vi "Main.vi"(8 "error in (no error)":errorcluster, 11 "ModuleAdmin":refnum<class "ModuleAdmin.lvclass">) -> ()   [LabVIEW 2018, in "SensorModule.lvlib"]
uses:
  SensorModule.lvlib
  <userlib>/NIST/ModuleAdminLib/ModuleAdmin/ModuleAdmin.lvclass
  C:/Program Files (x86)/National Instruments/LabVIEW 2018/user.lib/NIST/ModuleAdminLib/ModuleAdminBase/ModuleAdminBase.lvclass
  SensorPlugins/SensorBaseClass/SensorBase.lvclass
  C:/Program Files (x86)/National Instruments/LabVIEW 2018/user.lib/NIST/BaseClasses/BasePlugin_class/BasePlugin.lvclass
  PublicAPI/Arguments/Requests/clStopArgument.ctl
  <userlib>/NIST/ModuleAdminLib/ModuleAdmin/ModuleAdmin.lvclass/ModuleAdmin.ctl
  <userlib>/NIST/BaseClasses/BasePlugin_class/BasePlugin.lvclass/BasePlugin.ctl
  <vilib>/Utility/error.llb/DialogType.ctl
  <userlib>/NIST/ModuleAdminLib/ModuleAdmin/Accessors/Read ShowPanel_.vi
  <userlib>/NIST/ModuleAdminLib/ModuleAdmin/Accessors/Write ShowPanel_.vi
  <userlib>/NIST/BaseClasses/BasePlugin_class/Accessors/Write PluginIniFilePath.vi
  <userlib>/NIST/BaseClasses/BasePlugin_class/Accessors/Read PluginIniFilePath.vi
  <userlib>/NIST/ModuleAdminLib/ModuleAdmin/Accessors/Read CloneRegRef.vi
  <vilib>/Utility/error.llb/Error Cluster From Error Code.vi
  <vilib>/ErrorRing/Error Ring.xnode
  <userlib>/NIST/ModuleAdminLib/CloneRegistration/CloneRegistration.lvclass
  <userlib>/NIST/BaseClasses/Object_class/BaseObject.lvclass
  <userlib>/NIST/ModuleAdminLib/ModuleAdmin.lvlib
panel:
  out "error out":errorcluster
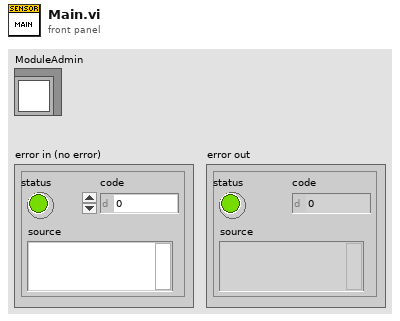
[diagram p1: front panel]
types:
  T1 = typedef "SensorModule.lvlib/clRequestEvents.ctl" = cluster{"StopRequest":refnum<user-event>, "PathToINI":refnum<user-event>, " LoadPlugin":refnum<user-event>, "ShowPanel":refnum<user-event>, "StartData":refnum<user-event>, "StopData":refnum<user-event>, "WriteConfig":refnum<user-event>, "ReadConfig":refnum<user-event>, "WriteEvtSignal":refnum<user-event>, "Configure":refnum<user-event>}
  T2 = typedef "SensorModule.lvlib/clBroadcastEvents.ctl" = cluster{"DidInit":refnum<user-event>, "StatusUpdate":refnum<user-event>, "ErrorReport":refnum<user-event>, "DidStop":refnum<user-event>, "PathToINI":refnum<user-event>, "SensorReport":refnum<user-event>, "SensorConfig":refnum<user-event>}
  T3 = typedef "SensorModule.lvlib/clStopArgument.ctl" = cluster{"Exit via Stop Module Req?":bool, "Wait for Module to stop?":bool, "ModuleAdmin":refnum<class "ModuleAdmin.lvclass">}
  T4 = enum32{"Invalid", "Standard", "Closed", "Hidden", "Minimized", "Maximized"}
  T5 = typedef "SensorModule.lvlib/clSensorData.ctl" = cluster{"SensorType":string, "SensorData":variant}
  T6 = typedef "DialogType.ctl" = u16
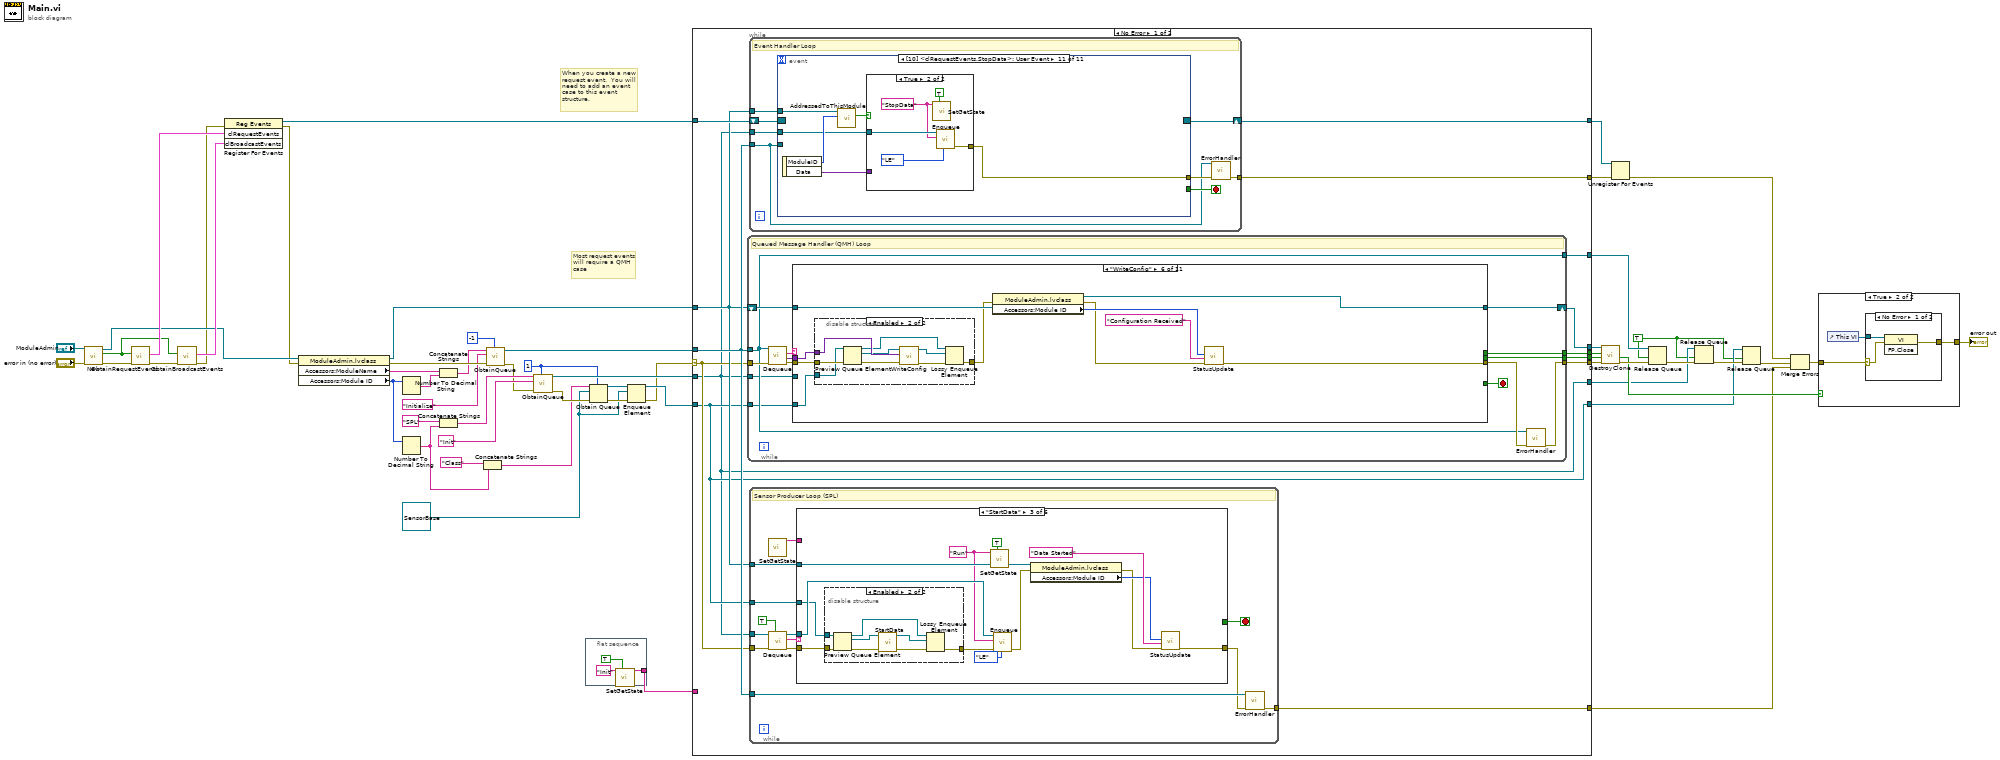
[diagram p0: block diagram]
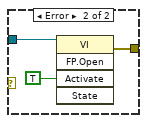
[diagram p3: hidden frame]
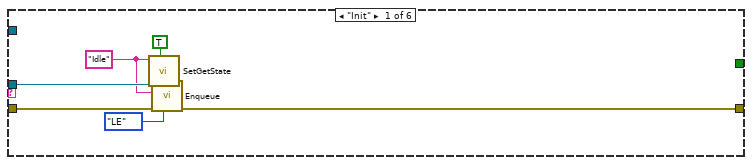
[diagram p4: hidden frame]
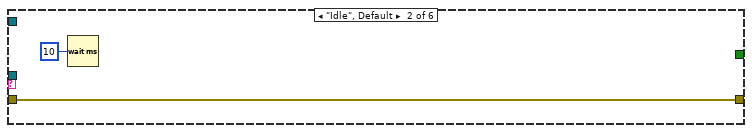
[diagram p5: hidden frame]
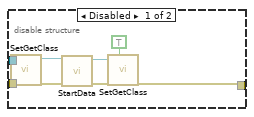
[diagram p6: hidden frame]
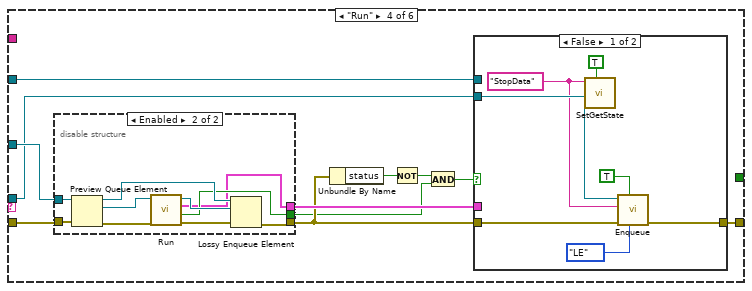
[diagram p7: hidden frame]
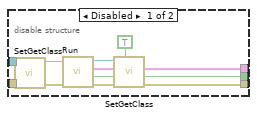
[diagram p8: hidden frame]
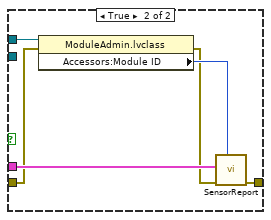
[diagram p9: hidden frame]
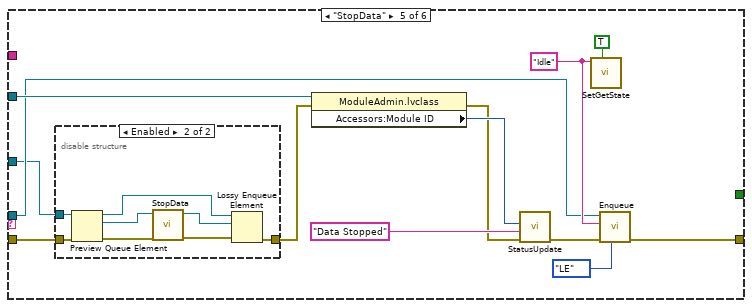
[diagram p10: hidden frame]
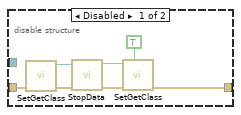
[diagram p11: hidden frame]
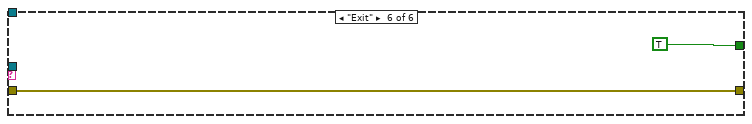
[diagram p12: hidden frame]
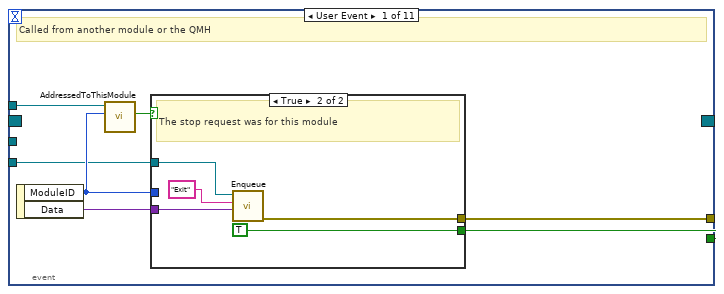
[diagram p13: hidden frame]
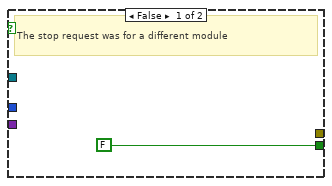
[diagram p14: hidden frame]
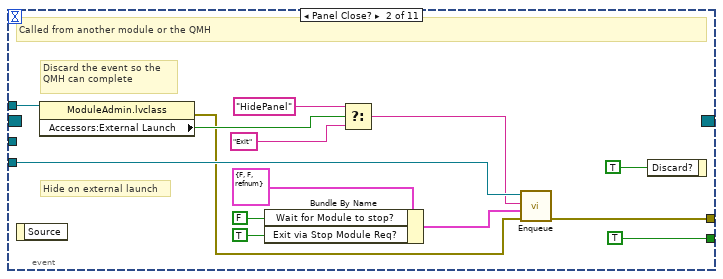
[diagram p15: hidden frame]
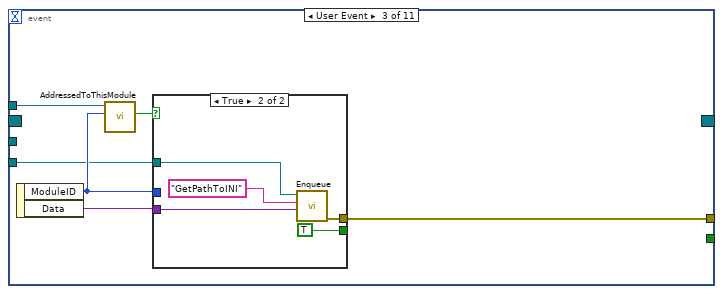
[diagram p16: hidden frame]
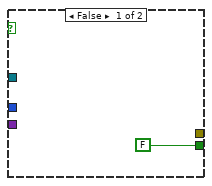
[diagram p17: hidden frame]
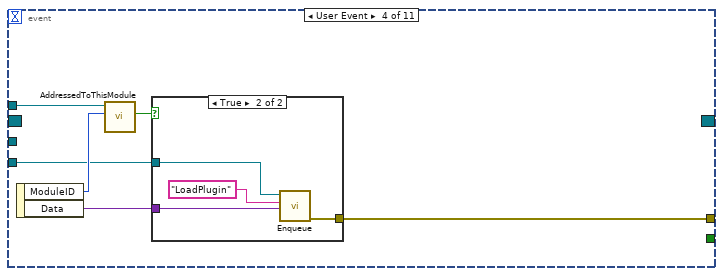
[diagram p18: hidden frame]
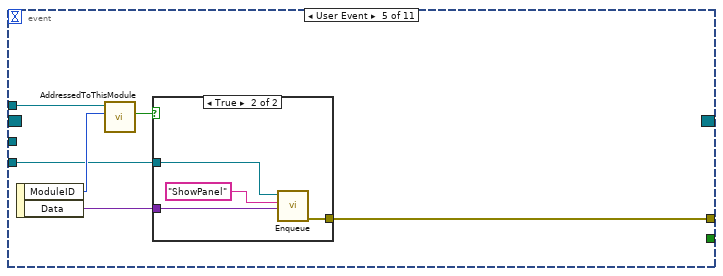
[diagram p20: hidden frame]
diagram:
  w2 = TRUE ("force destroy? (F)")
  w11 = refnum<class "SensorBase.lvclass"> refnum ("MyPlugins.lvlib:MyPluginsBase.lvclass")
  w1 = 1 ("Queue size (-1, unlimited)")
  # "Most request events\nwill require a QMH\ncase"
  # "When you create a new request event.  You will need to add an event case to this event structure."
  n1 = call <userlib>:"New.vi"("error in (no error)"="error in (no error)", "ModuleAdmin"="ModuleAdmin") -> ("error out"=w53:errorcluster, "First?"=w49:bool, "ModuleAdmin"=w34:refnum<class "ModuleAdmin.lvclass">)  [unwired: 6 in, 1 out]
  n2 = call "ObtainRequestEvents.vi"("error in (no error)"=w53, "CreateNew (F)"=w49) -> ("error out"=w48:errorcluster, "clRequestEvents"=w52:T1)  [unwired: 8 in]
  n3 = call "ObtainBroadcastEvents.vi"("error in (no error)"=w48, "CreateNew? (F)"=w49) -> ("error out"=w21:errorcluster, "clBroadcastEvents"=w47:T2)  [unwired: 8 in]
  n4 = register-events(error in=w21, w52, w47) -> (reference out=w46:refnum<event-registration>, error out=w20:errorcluster)  [unwired: 1 in]
  n5 = property class="ModuleAdmin.lvclass"(reference=w34, error in=w20) -> (reference out=w8:refnum<class "ModuleAdmin.lvclass">, error out=w36:errorcluster, "Accessors:ModuleName"=w32:string, "Accessors:Module ID"=w24:i32)
  n6 = Number To Decimal String(number=w24) -> (decimal integer string=w31:string)  [unwired: 1 in]
  n7 = Number To Decimal String(number=w24) -> (decimal integer string=w15:string)  [unwired: 1 in]
  n8 = Concatenate Strings(w32, w31) -> (w30:string)
  n9 = Concatenate Strings("SPL" ("Initial Message"), w15) -> (w26:string)
  n10 = Concatenate Strings("Class" ("Initial Message"), w15) -> (w14:string)
  n11 = call "ObtainQueue.vi"("Queue size (-1, unlimited)"=-1, "error in (no error)"=w36, "Initial Message"="Initialize", "Queue Name"=w30) -> ("error out"=w25:errorcluster, "MessageQueue"=w51:refnum<queue>)  [unwired: 6 in]
  n12 = call "ObtainQueue.vi"("Queue size (-1, unlimited)"=w1, "error in (no error)"=w25, "Initial Message"="Init", "Queue Name"=w26) -> ("error out"=w18:errorcluster, "MessageQueue"=w22:refnum<queue>)  [unwired: 6 in]
  n13 = flat-sequence {
    tunnel: [w56] -> w9
    frame #0 {
      n14 = call "SetGetState.vi"("Set (f)"=TRUE, "State In"="Init") -> ("State Out"=w56:string)  [unwired: 9 in]
    }
  }
  n15 = Obtain Queue(max queue size (-1, unlimited)=w1, name (unnamed)=w14, element data type=w11, error in (no error)=w18) -> (queue out=w13:refnum<queue>, error out=w17:errorcluster)  [unwired: 1 in, 1 out]
  n16 = Enqueue Element(queue=w13, element=w11, error in (no error)=w17) -> (queue out=w12:refnum<queue>, error out=w10:errorcluster)  [unwired: 1 in, 1 out]
  n17 = case shown="No Error" w10 {
    selector: w10 -> [w61 w618]
    tunnel: w51 -> [w65 w614]
    tunnel: w8 -> [w63 w615]
    tunnel: [w72 w616] -> w45
    tunnel: [w71 w614] -> w50
    tunnel: w46 -> [w70 w610]
    tunnel: [w69 w613] -> w43
    tunnel: [w68 _] -> w42
    tunnel: [w67 _] -> w41
    tunnel: [w66 _] -> w39
    tunnel: [w64 _] -> w19
    tunnel: [w62 w610] -> w38
    tunnel: w22 -> [w59 w607]
    tunnel: w12 -> [w60 w606]
    tunnel: w9 -> [_ _]
    tunnel: [w59 w607] -> w4
    tunnel: [w60 w606] -> w3
    frame No Error {
      n18 = while {
        tunnel: w65 -> [w321]
        tunnel: w61 -> [w330]
        tunnel: [w323] -> w72
        tunnel: [w321] -> w71
        tunnel: [w325] -> w68
        tunnel: [w324] -> w67
        shift-right: [w320] -> w69
        shift-left: w63 -> [w326]
        tunnel: w60 -> [w319]
        tunnel: w59 -> [w318]
        stop <- w331 stop-if-true
        # "Queued Message Handler (QMH) Loop"
        n19 = call "Dequeue.vi"("error in (no error)"=w330, "MessageQueue"=w321) -> ("error out"=w329:errorcluster, "Message Data"=w327:variant, "Message"=w328:string)  [unwired: 6 in, 1 out]
        n20 = case shown="\"WriteConfig\"" w328 {
          selector: w328 -> [_ _ _ _ _ _ _ _ _ _ w594]
          tunnel: [_ _ _ _ _ _ _ _ w562 _ _] -> w331
          tunnel: w326 -> [w354 w371 w378 w448 w463 w493 w517 w539 w563 w572 w597]
          tunnel: [w343 w365 w379 w449 w462 w491 w513 w537 w557 w573 w588] -> w322
          tunnel: w329 -> [w332 w374 w388 w446 w464 w487 w519 w533 w559 w570 w591]
          tunnel: w327 -> [_ w373 w390 _ _ w488 _ w534 w567 w580 _]
          tunnel: [_ _ _ _ _ _ _ _ w565 _ _] -> w325
          tunnel: [_ _ _ _ _ _ _ _ w564 _ _] -> w324
          tunnel: [w336 w370 w376 w445 w463 w492 w512 w538 w563 w568 w592] -> w320
          tunnel: w319 -> [_ _ w375 w442 w461 w484 w509 w530 _ _ _]
          tunnel: w318 -> [_ _ _ _ _ _ _ _ w561 _ _]
          frame "Initialize" {
            # "Initialize is always called after ObtainQueue.vi is run"
            n21 = property class="ModuleAdmin.lvclass"(reference=w354, error in=w332) -> (reference out=w341:refnum<class "ModuleAdmin.lvclass">, error out=w351:errorcluster, "Accessors:Module ID"=w333:i32, "Accessors:ShowPanel_"=w339:bool, "Accessors:External Launch"=w338:bool, "Accessors:ModuleName"=w340:string)
            n22 = call "SetGetClass.vi"("Set (f)"=TRUE, "Class In"=refnum<class "SensorBase.lvclass"> refnum ("MyPlugins.lvlib:MyPluginsBase.lvclass")) -> ()  [unwired: 9 in, 1 out]
            n23 = Compound Arithmetic op=OR(w339, invert w338) -> (w337:bool)
            n24 = Select(t=T4."Standard" ("Front Panel Window:State"), s=w337, f=T4."Hidden" ("Front Panel Window:State")) -> (s? t:f=w347:T4)
            n25 = invoke class="VI" method="FP.Open"(error in=w351, "State"=w347) -> (error out=w350:errorcluster)  [unwired: 3 in, 4 out]
            n26 = call <userlib>:"ModuleName.vi"("Name"=w340, "ModuleID"=w333) -> ("ModuleName"=w346:string)  [unwired: 9 in]
            n27 = property class="VI"(error in=w350, "Front Panel.Title"=w346) -> (reference out=w353:refnum<vi>, error out=w352:errorcluster)  [unwired: 1 in]
            n28 = invoke class="VI" method="FP.Center"(reference=w353, error in=w352) -> (error out=w342:errorcluster)  [unwired: 1 in, 2 out]
            n29 = case shown="True" w338 {
              tunnel: [w355 w361] -> w344
              tunnel: [w356 w358] -> w336
              tunnel: w342 -> [w355 w360]
              tunnel: w341 -> [w356 w357]
              frame False {
              }
              frame True {
                n30 = call <userlib>:"WaitOnModuleSync.vi"("error in (no error)"=w360, "ModuleAdmin"=w357) -> ("error out"=w362:errorcluster, "ModuleAdmin"=w359:refnum<class "ModuleAdmin.lvclass">)  [unwired: 8 in]
                n31 = call <userlib>:"WaitOnEventSync.vi"("error in (no error)"=w362, "ModuleAdmin"=w359) -> ("error out"=w361:errorcluster, "ModuleAdmin"=w358:refnum<class "ModuleAdmin.lvclass">)  [unwired: 8 in]
              }
            }
            n32 = call "DidInit.vi"("Init?"=TRUE, "error in (no error)"=w344, "ModuleAdmin"=w336) -> ("error out"=w343:errorcluster)  [unwired: 8 in]
          }
          frame "ShowPanel" {
            n33 = Variant To Data(error in=w374, type=TRUE, Variant=w373) -> (data=w367:bool, error out=w364:errorcluster)
            n34 = property class="ModuleAdmin.lvclass"(reference=w371, error in=w364, "Accessors:ShowPanel_"=w367) -> (reference out=w370:refnum<class "ModuleAdmin.lvclass">, error out=w363:errorcluster)
            n35 = Select(t=T4."Standard" ("Front Panel Window:State"), s=w367, f=T4."Hidden" ("Front Panel Window:State")) -> (s? t:f=w366:T4)
            n36 = property class="VI"(error in=w363, "FP.State"=w366) -> (error out=w365:errorcluster)  [unwired: 1 in, 1 out]
          }
          frame "LoadPlugin" {
            n37 = Variant To Data(error in=w388, type=path "", Variant=w390) -> (data=w377:path, error out=w387:errorcluster)
            n38 = Current VI's Path() -> (path=w385:path)
            n39 = call <userlib>:"GetPathToClass.vi"("error in (no error)"=w387, "configuration file path"=w377) -> ("error IO"=w383:errorcluster, "PathToClass"=w386:path)  [unwired: 8 in]
            n40 = Build Path(base path=w385, name or relative path=w386) -> (appended path=w384:path)
            n41 = call <vilib>:"Check if File or Folder Exists.vi"("error in (no error)"=w383, "path"=w384) -> ("error out"=w380:errorcluster, "file or folder exists?"=w382:bool, "dup path"=w381:path)  [unwired: 7 in]
            n42 = case shown="False" w382 {
              tunnel: w381 -> [w393 w404]
              tunnel: w380 -> [_ w416]
              tunnel: [w392 w407] -> w379
              tunnel: w378 -> [w391 w412]
              tunnel: w377 -> [_ w410]
              tunnel: [w391 w409] -> w376
              tunnel: w375 -> [_ w402]
              frame False {
                n43 = Path To String(path=w393) -> (string=w394:string)
                n44 = xnode "Error Ring"("parameter 0"=w394) -> ("error out"=w392:errorcluster)
              }
              frame True {
                n45 = disable-structure shown="Enabled" {
                  disable-tunnel: w416 -> [w427 w435]
                  disable-tunnel: w410 -> [w423 w439]
                  disable-tunnel: [w418 w429] -> w406
                  disable-tunnel: w404 -> [w417 w436]
                  disable-tunnel: [w417 w436] -> w403
                  disable-tunnel: w402 -> [_ w432]
                  frame Disabled {
                    n46 = call-dynamic "LoadClassFromFile.vi"("error in (no error)"=w427, "class path"=w417, "reference in"=refnum<class "SensorBase.lvclass"> refnum ("MyPlugins.lvlib:MyPluginsBase.lvclass")) -> ("error out"=w424:errorcluster, "reference out"=w425:refnum<class "SensorBase.lvclass">)  [unwired: 7 in]
                    n47 = property class="SensorBase.lvclass"(reference=w425, error in=w424, "Accessors:PluginIniFilePath"=w423) -> (reference out=w421:refnum<class "SensorBase.lvclass">, error out=w419:errorcluster)
                    n48 = call-dynamic "DefaultFromIni.vi"("error in (no error)"=w419, "SensorBase in"=w421) -> ("error out"=w418:errorcluster, "SensorBase out"=w420:refnum<class "SensorBase.lvclass">)  [unwired: 8 in]
                    n49 = call "SetGetClass.vi"("Set (f)"=TRUE, "Class In"=w420) -> ()  [unwired: 9 in, 1 out]
                  }
                  frame Enabled {
                    n50 = Preview Queue Element(queue=w432, error in (no error)=w435) -> (queue out=w428:refnum<queue>, element=w433:refnum<class "SensorBase.lvclass">, error out=w434:errorcluster)  [unwired: 1 in, 1 out]
                    n51 = call-dynamic "LoadClassFromFile.vi"("error in (no error)"=w434, "class path"=w436, "reference in"=w433) -> ("error out"=w440:errorcluster, "reference out"=w441:refnum<class "SensorBase.lvclass">)  [unwired: 7 in]
                    n52 = property class="SensorBase.lvclass"(reference=w441, error in=w440, "Accessors:PluginIniFilePath"=w439) -> (reference out=w438:refnum<class "SensorBase.lvclass">, error out=w437:errorcluster)
                    n53 = call-dynamic "DefaultFromIni.vi"("error in (no error)"=w437, "SensorBase in"=w438) -> ("error out"=w430:errorcluster, "SensorBase out"=w431:refnum<class "SensorBase.lvclass">)  [unwired: 8 in]
                    n54 = Lossy Enqueue Element(queue=w428, element=w431, error in (no error)=w430) -> (error out=w429:errorcluster)  [unwired: 3 out]
                  }
                }
                n55 = Path To String(path=w403) -> (string=w414:string)
                n56 = Format Into String(format string="Plugin %s loaded ", error in=w406, w414) -> (resulting string=w413:string, error out=w405:errorcluster)  [unwired: 1 in]
                n57 = property class="ModuleAdmin.lvclass"(reference=w412, error in=w405) -> (reference out=w409:refnum<class "ModuleAdmin.lvclass">, error out=w408:errorcluster, "Accessors:Module ID"=w411:i32)
                n58 = call "StatusUpdate.vi"("error in (no error)"=w408, "Status"=w413, "ModuleID"=w411) -> ("error out"=w407:errorcluster)  [unwired: 8 in]
              }
            }
          }
          frame "GetPathToINI" {
            n59 = disable-structure shown="Enabled" {
              disable-tunnel: [w454 w459] -> w447
              disable-tunnel: w446 -> [w453 w458]
              disable-tunnel: [w451 w460] -> w444
              disable-tunnel: w442 -> [_ w456]
              frame Disabled {
                n60 = call "SetGetClass.vi"() -> ("Class Out"=w452:refnum<class "SensorBase.lvclass">)  [unwired: 11 in]
                n61 = property class="SensorBase.lvclass"(reference=w452, error in=w453) -> (error out=w451:errorcluster, "Accessors:PluginIniFilePath"=w454:path)  [unwired: 1 out]
              }
              frame Enabled {
                n62 = Preview Queue Element(queue=w456, error in (no error)=w458) -> (element=w455:refnum<class "SensorBase.lvclass">, error out=w457:errorcluster)  [unwired: 1 in, 2 out]
                n63 = property class="SensorBase.lvclass"(reference=w455, error in=w457) -> (error out=w460:errorcluster, "Accessors:PluginIniFilePath"=w459:path)  [unwired: 1 out]
              }
            }
            n64 = property class="ModuleAdmin.lvclass"(reference=w448, error in=w444) -> (reference out=w445:refnum<class "ModuleAdmin.lvclass">, error out=w443:errorcluster, "Accessors:Module ID"=w450:i32)
            n65 = call "PathToINIBroadcast.vi"("error in (no error)"=w443, "PathToINI"=w447, "ModuleID"=w450) -> ("error out"=w449:errorcluster)  [unwired: 8 in]
          }
          frame "Configure" {
            n66 = disable-structure shown="Enabled" {
              disable-tunnel: w464 -> [w468 w478]
              disable-tunnel: [w465 w475] -> w462
              disable-tunnel: w461 -> [_ w471]
              frame Disabled {
                n67 = call "SetGetClass.vi"() -> ("Class Out"=w469:refnum<class "SensorBase.lvclass">)  [unwired: 11 in]
                n68 = call-dynamic "ConfigureDlg.vi"("error in (no error)"=w468, "PmuBase in"=w469) -> ("error out"=w465:errorcluster, "PmuBase out"=w467:refnum<class "SensorBase.lvclass">)  [unwired: 7 in, 1 out]
                n69 = call "SetGetClass.vi"("Set (f)"=TRUE, "Class In"=w467) -> ()  [unwired: 9 in, 1 out]
              }
              frame Enabled {
                n70 = Preview Queue Element(queue=w471, error in (no error)=w478) -> (queue out=w473:refnum<queue>, element=w474:refnum<class "SensorBase.lvclass">, error out=w477:errorcluster)  [unwired: 1 in, 1 out]
                n71 = call-dynamic "ConfigureDlg.vi"("error in (no error)"=w477, "PmuBase in"=w474) -> ("error out"=w476:errorcluster, "Changed"=w472:bool, "PmuBase out"=w470:refnum<class "SensorBase.lvclass">)  [unwired: 7 in]
                n72 = case shown="True" w472 {
                  tunnel: w476 -> [w479 w483]
                  tunnel: [w479 w482] -> w475
                  tunnel: w473 -> [_ w481]
                  tunnel: w470 -> [_ w480]
                  frame False {
                  }
                  frame True {
                    n73 = Lossy Enqueue Element(queue=w481, element=w480, error in (no error)=w483) -> (error out=w482:errorcluster)  [unwired: 3 out]
                  }
                }
              }
            }
          }
          frame "WriteConfig" {
            n74 = disable-structure shown="Enabled" {
              disable-tunnel: w488 -> [w498 w503]
              disable-tunnel: w487 -> [w497 w508]
              disable-tunnel: [w494 w505] -> w486
              disable-tunnel: w484 -> [_ w502]
              frame Disabled {
                n75 = call "SetGetClass.vi"() -> ("Class Out"=w499:refnum<class "SensorBase.lvclass">)  [unwired: 11 in]
                n76 = call-dynamic "WriteConfig.vi"("error in (no error)"=w497, "Config"=w498, "SensorBase in"=w499) -> ("error out"=w494:errorcluster, "SensorBase out"=w496:refnum<class "SensorBase.lvclass">)  [unwired: 7 in]
                n77 = call "SetGetClass.vi"("Set (f)"=TRUE, "Class In"=w496) -> ()  [unwired: 9 in, 1 out]
              }
              frame Enabled {
                n78 = Preview Queue Element(queue=w502, error in (no error)=w508) -> (queue out=w501:refnum<queue>, element=w500:refnum<class "SensorBase.lvclass">, error out=w507:errorcluster)  [unwired: 1 in, 1 out]
                n79 = call-dynamic "WriteConfig.vi"("error in (no error)"=w507, "Config"=w503, "SensorBase in"=w500) -> ("error out"=w506:errorcluster, "SensorBase out"=w504:refnum<class "SensorBase.lvclass">)  [unwired: 7 in]
                n80 = Lossy Enqueue Element(queue=w501, element=w504, error in (no error)=w506) -> (error out=w505:errorcluster)  [unwired: 3 out]
              }
            }
            n81 = property class="ModuleAdmin.lvclass"(reference=w493, error in=w486) -> (reference out=w492:refnum<class "ModuleAdmin.lvclass">, error out=w485:errorcluster, "Accessors:Module ID"=w490:i32)
            n82 = call "StatusUpdate.vi"("error in (no error)"=w485, "Status"="Configuration Received", "ModuleID"=w490) -> ("error out"=w491:errorcluster)  [unwired: 8 in]
          }
          frame "ReadConfig" {
            n83 = disable-structure shown="Enabled" {
              disable-tunnel: w519 -> [w522 w527]
              disable-tunnel: [w521 w529] -> w511
              disable-tunnel: [w520 w528] -> w518
              disable-tunnel: w509 -> [_ w524]
              frame Disabled {
                n84 = call "SetGetClass.vi"() -> ("Class Out"=w523:refnum<class "SensorBase.lvclass">)  [unwired: 11 in]
                n85 = call-dynamic "ReadConfig.vi"("error in (no error)"=w522, "SensorBase in"=w523) -> ("error out"=w521:errorcluster, "Config"=w520:variant)  [unwired: 7 in, 1 out]
              }
              frame Enabled {
                n86 = Preview Queue Element(queue=w524, error in (no error)=w527) -> (element=w525:refnum<class "SensorBase.lvclass">, error out=w526:errorcluster)  [unwired: 1 in, 2 out]
                n87 = call-dynamic "ReadConfig.vi"("error in (no error)"=w526, "SensorBase in"=w525) -> ("error out"=w529:errorcluster, "Config"=w528:variant)  [unwired: 7 in, 1 out]
              }
            }
            n88 = property class="ModuleAdmin.lvclass"(reference=w517, error in=w511) -> (reference out=w512:refnum<class "ModuleAdmin.lvclass">, error out=w510:errorcluster, "Accessors:Module ID"=w516:i32)
            n89 = call "SensorConfig.vi"("ModuleID"=w516, "error in (no error)"=w510, "Config"=w518) -> ("error out"=w515:errorcluster)  [unwired: 8 in]
            n90 = call "StatusUpdate.vi"("error in (no error)"=w515, "Status"="Config Transmitted", "ModuleID"=w516) -> ("error out"=w513:errorcluster)  [unwired: 8 in]
          }
          frame "WriteEvtSignal" {
            n91 = disable-structure shown="Enabled" {
              disable-tunnel: w534 -> [w544 w554]
              disable-tunnel: w533 -> [w543 w553]
              disable-tunnel: [w540 w549] -> w532
              disable-tunnel: w530 -> [_ w552]
              frame Disabled {
                n92 = call "SetGetClass.vi"() -> ("Class Out"=w545:refnum<class "SensorBase.lvclass">)  [unwired: 11 in]
                n93 = call-dynamic "WriteEvtSignal.vi"("error in (no error)"=w543, "EvtSignal"=w544, "SensorBase in"=w545) -> ("error out"=w540:errorcluster, "SensorBase out"=w542:refnum<class "SensorBase.lvclass">)  [unwired: 7 in]
                n94 = call "SetGetClass.vi"("Set (f)"=TRUE, "Class In"=w542) -> ()  [unwired: 9 in, 1 out]
              }
              frame Enabled {
                n95 = Preview Queue Element(queue=w552, error in (no error)=w553) -> (queue out=w546:refnum<queue>, element=w550:refnum<class "SensorBase.lvclass">, error out=w551:errorcluster)  [unwired: 1 in, 1 out]
                n96 = call-dynamic "WriteEvtSignal.vi"("error in (no error)"=w551, "EvtSignal"=w554, "SensorBase in"=w550) -> ("error out"=w548:errorcluster, "SensorBase out"=w547:refnum<class "SensorBase.lvclass">)  [unwired: 7 in]
                n97 = Enqueue Element(queue=w546, element=w547, error in (no error)=w548) -> (error out=w549:errorcluster)  [unwired: 1 in, 2 out]
              }
            }
            n98 = property class="ModuleAdmin.lvclass"(reference=w539, error in=w532) -> (reference out=w538:refnum<class "ModuleAdmin.lvclass">, error out=w531:errorcluster, "Accessors:Module ID"=w536:i32)
            n99 = call "StatusUpdate.vi"("error in (no error)"=w531, "Status"="Waveform Received", "ModuleID"=w536) -> ("error out"=w537:errorcluster)  [unwired: 8 in]
          }
          frame "Exit" {
            w556 = "Exit" ("State In")
            w562 = TRUE
            # "Called by the StopRequest event handler case"
            n100 = control-ref of="This VI"() -> (w566:refnum<vi>)
            n101 = call "HandleExit.vi"("error in (no error)"=w559, "VI Refnum"=w566, "StopArgument"=w567, "ModuleAdmin"=w563) -> ("error out"=w558:errorcluster, "Exit via Stop Module Req?"=w564:bool, "WaitForStop?"=w565:bool)  [unwired: 5 in]
            n102 = call "Enqueue.vi"("Enum"=enum16{"Else", "LE"}."LE", "Priority (F)"=TRUE, "error in (no error)"=w558, "Message"=w556, "MessageQueue"=w561) -> ("error out"=w557:errorcluster)  [unwired: 5 in, 1 out]
            n103 = call "SetGetState.vi"("Set (f)"=w562, "State In"=w556) -> ()  [unwired: 9 in, 1 out]
          }
          frame "Error" {
            n104 = property class="ModuleAdmin.lvclass"(reference=w572, error in=w570) -> (reference out=w571:refnum<class "ModuleAdmin.lvclass">, error out=w569:errorcluster, "Accessors:External Launch"=w576:bool, "Accessors:Module ID"=w574:i32)
            n105 = Variant To Data(error in=w569, type=errorcluster {"status"=FALSE, "code"=0, "source"=""} ("error constant"), Variant=w580) -> (data=w575:errorcluster, error out=w578:errorcluster)
            n106 = call "ReportError.vi"("error in (no error)"=w578, "ErrorReported"=w575, "ModuleID"=w574) -> ("error out"=w577:errorcluster)  [unwired: 8 in]
            n107 = case shown="False" w576 {
              tunnel: w577 -> [w585 w587]
              tunnel: w575 -> [w584 _]
              tunnel: [w583 w587] -> w573
              tunnel: w571 -> [w582 w586]
              tunnel: [w581 w586] -> w568
              frame False {
                # "Todo:  Add an event to ask the user\nIf the module should stop or continue"
                # "Stand alone: now, force an exit"
                n108 = call "StopRequest.vi"("error in (no error)"=w585, "ModuleAdminIn"=w582) -> ("error out"=w583:errorcluster, "ModuleAdminOut"=w581:refnum<class "ModuleAdmin.lvclass">)  [unwired: 7 in, 1 out]
                n109 = call <vilib>:"Simple Error Handler.vi"("error in (no error)"=w584) -> ()  [unwired: 4 in, 5 out]
              }
              frame True {
                # "Externally launched modules only broadcast the error msg"
              }
            }
          }
          frame Default {
            # "Called only if a message was queued and no QMH case was created"
            n110 = property class="ModuleAdmin.lvclass"(reference=w597, error in=w591) -> (reference out=w592:refnum<class "ModuleAdmin.lvclass">, error out=w589:errorcluster, "Accessors:Module ID"=w596:i32, "Accessors:ModuleName"=w593:string)
            n111 = call <userlib>:"ModuleName.vi"("Name"=w593, "ModuleID"=w596) -> ("ModuleName"=w595:string)  [unwired: 9 in]
            n112 = xnode "Error Ring"("parameter 0"=w594, "parameter 1"=w595) -> ("error out"=w590:errorcluster)
            n113 = Merge Errors(w589, w590) -> (w588:errorcluster)
          }
        }
        n114 = call "ErrorHandler.vi"("error in (no error)"=w322, "MessageQueue"=w321) -> ("error out"=w323:errorcluster)  [unwired: 8 in, 1 out]
      }
      n115 = while {
        tunnel: w65 -> [w190]
        shift-right: [w194] -> w62
        shift-left: w70 -> [w195]
        tunnel: w63 -> [w193]
        tunnel: [w191] -> w66
        tunnel: w59 -> [w189]
        stop <- w196 stop-if-true
        # "Event Handler Loop"
        n116 = event shown="[10] <clRequestEvents.StopData>: User Event" {
          selector: w195 -> [_ _ _ _ _ _ _ _ _ _ _]
          dyn-events: [_ _ _ _ _ _ _ _ _ _ _] -> w194
          timeout: _ -> [_ _ _ _ _ _ _ _ _ _ _]
          tunnel: w190 -> [w200 w223 w226 w237 w247 w257 w267 w277 w287 _ _]
          tunnel: [w199 TRUE _ _ _ _ _ _ _ _ _] -> w196
          tunnel: w193 -> [w203 w217 w225 w241 w251 w261 w271 w281 w291 w301 w312]
          tunnel: [w198 w221 w224 w238 w248 w258 w268 w278 w288 w297 w308] -> w192
          tunnel: w189 -> [_ _ _ _ _ _ _ _ _ w296 w307]
          event User Event {
            # "Called from another module or the QMH"
            n117 = event-data() -> ("ModuleID"=w201:i32, "Data"=w197:variant)  [unwired: 1 in]
            n118 = call <userlib>:"AddressedToThisModule.vi"("ModuleID"=w201, "ModuleAdmin"=w203) -> ("AddressedToThisInstance?"=w202:bool)  [unwired: 8 in, 1 out]
            n119 = case shown="True" w202 {
              tunnel: w201 -> [_ _]
              tunnel: w200 -> [_ w209]
              tunnel: [FALSE TRUE] -> w199
              tunnel: [_ w207] -> w198
              tunnel: w197 -> [_ w205]
              frame False {
                # "The stop request was for a different module"
              }
              frame True {
                # "The stop request was for this module"
                n120 = call "Enqueue.vi"("Message Data"=w205, "Message"="Exit", "MessageQueue"=w209) -> ("error out"=w207:errorcluster)  [unwired: 7 in, 1 out]
              }
            }
          }
          event Panel Close? {
            # "Hide on external launch"
            # "Discard the event so the QMH can complete"
            # "Called from another module or the QMH"
            n121 = event-data() -> ()  [unwired: 1 in, 1 out]
            n122 = property class="ModuleAdmin.lvclass"(reference=w217) -> (error out=w210:errorcluster, "Accessors:External Launch"=w212:bool)  [unwired: 1 in, 1 out]
            n123 = Bundle By Name(cluster=T3 {"Exit via Stop Module Req?"=FALSE, "Wait for Module to stop?"=FALSE, "ModuleAdmin"=refnum} ("Stop Argument"), "Wait for Module to stop?"=FALSE, "Exit via Stop Module Req?"=TRUE) -> (w218:T3)
            n124 = Select(t="HidePanel", s=w212, f="Exit" ("Message")) -> (s? t:f=w214:string)
            n125 = call "Enqueue.vi"("error in (no error)"=w210, "Message Data"=w218, "Message"=w214, "MessageQueue"=w223) -> ("error out"=w221:errorcluster)  [unwired: 6 in, 1 out]
            n126 = event-data("Discard?"=TRUE) -> ()  [unwired: 1 in, 1 out]
          }
          event User Event {
            n127 = event-data() -> ("ModuleID"=w227:i32, "Data"=w228:variant)  [unwired: 1 in]
            n128 = call <userlib>:"AddressedToThisModule.vi"("ModuleID"=w227, "ModuleAdmin"=w225) -> ("AddressedToThisInstance?"=w229:bool)  [unwired: 8 in, 1 out]
            n129 = case shown="True" w229 {
              tunnel: w227 -> [_ _]
              tunnel: w226 -> [_ w235]
              tunnel: [FALSE TRUE] -> _
              tunnel: [_ w233] -> w224
              tunnel: w228 -> [_ w231]
              frame False {
                # "The stop request was for a different module"
              }
              frame True {
                # "The stop request was for this module"
                n130 = call "Enqueue.vi"("Message Data"=w231, "Message"="GetPathToINI", "MessageQueue"=w235) -> ("error out"=w233:errorcluster)  [unwired: 7 in, 1 out]
              }
            }
          }
          event User Event {
            n131 = event-data() -> ("ModuleID"=w240:i32, "Data"=w236:variant)  [unwired: 1 in]
            n132 = call <userlib>:"AddressedToThisModule.vi"("ModuleID"=w240, "ModuleAdmin"=w241) -> ("AddressedToThisInstance?"=w239:bool)  [unwired: 8 in, 1 out]
            n133 = case shown="True" w239 {
              tunnel: [_ w242] -> w238
              tunnel: w237 -> [_ w245]
              tunnel: w236 -> [_ w243]
              frame False {
              }
              frame True {
                n134 = call "Enqueue.vi"("Message Data"=w243, "Message"="LoadPlugin", "MessageQueue"=w245) -> ("error out"=w242:errorcluster)  [unwired: 7 in, 1 out]
              }
            }
          }
          event User Event {
            n135 = event-data() -> ("ModuleID"=w250:i32, "Data"=w246:variant)  [unwired: 1 in]
            n136 = call <userlib>:"AddressedToThisModule.vi"("ModuleID"=w250, "ModuleAdmin"=w251) -> ("AddressedToThisInstance?"=w249:bool)  [unwired: 8 in, 1 out]
            n137 = case shown="True" w249 {
              tunnel: [_ w252] -> w248
              tunnel: w247 -> [_ w255]
              tunnel: w246 -> [_ w253]
              frame False {
              }
              frame True {
                n138 = call "Enqueue.vi"("Message Data"=w253, "Message"="ShowPanel", "MessageQueue"=w255) -> ("error out"=w252:errorcluster)  [unwired: 7 in, 1 out]
              }
            }
          }
          event User Event {
            n139 = event-data() -> ("ModuleID"=w260:i32, "Data"=w256:variant)  [unwired: 1 in]
            n140 = call <userlib>:"AddressedToThisModule.vi"("ModuleID"=w260, "ModuleAdmin"=w261) -> ("AddressedToThisInstance?"=w259:bool)  [unwired: 8 in, 1 out]
            n141 = case shown="True" w259 {
              tunnel: [_ w262] -> w258
              tunnel: w257 -> [_ w265]
              tunnel: w256 -> [_ w263]
              frame False {
              }
              frame True {
                n142 = call "Enqueue.vi"("Message Data"=w263, "Message"="Configure", "MessageQueue"=w265) -> ("error out"=w262:errorcluster)  [unwired: 7 in, 1 out]
              }
            }
          }
          event User Event {
            n143 = event-data() -> ("ModuleID"=w270:i32, "Data"=w266:variant)  [unwired: 1 in]
            n144 = call <userlib>:"AddressedToThisModule.vi"("ModuleID"=w270, "ModuleAdmin"=w271) -> ("AddressedToThisInstance?"=w269:bool)  [unwired: 8 in, 1 out]
            n145 = case shown="True" w269 {
              tunnel: [_ w272] -> w268
              tunnel: w267 -> [_ w275]
              tunnel: w266 -> [_ w273]
              frame False {
              }
              frame True {
                n146 = call "Enqueue.vi"("Message Data"=w273, "Message"="WriteConfig", "MessageQueue"=w275) -> ("error out"=w272:errorcluster)  [unwired: 7 in, 1 out]
              }
            }
          }
          event User Event {
            n147 = event-data() -> ("ModuleID"=w280:i32, "Data"=w276:variant)  [unwired: 1 in]
            n148 = call <userlib>:"AddressedToThisModule.vi"("ModuleID"=w280, "ModuleAdmin"=w281) -> ("AddressedToThisInstance?"=w279:bool)  [unwired: 8 in, 1 out]
            n149 = case shown="True" w279 {
              tunnel: [_ w282] -> w278
              tunnel: w277 -> [_ w285]
              tunnel: w276 -> [_ w283]
              frame False {
              }
              frame True {
                n150 = call "Enqueue.vi"("Message Data"=w283, "Message"="ReadConfig", "MessageQueue"=w285) -> ("error out"=w282:errorcluster)  [unwired: 7 in, 1 out]
              }
            }
          }
          event User Event {
            n151 = event-data() -> ("ModuleID"=w290:i32, "Data"=w286:variant)  [unwired: 1 in]
            n152 = call <userlib>:"AddressedToThisModule.vi"("ModuleID"=w290, "ModuleAdmin"=w291) -> ("AddressedToThisInstance?"=w289:bool)  [unwired: 8 in, 1 out]
            n153 = case shown="True" w289 {
              tunnel: [_ w292] -> w288
              tunnel: w287 -> [_ w295]
              tunnel: w286 -> [_ w293]
              frame False {
              }
              frame True {
                n154 = call "Enqueue.vi"("Message Data"=w293, "Message"="WriteEvtSignal", "MessageQueue"=w295) -> ("error out"=w292:errorcluster)  [unwired: 7 in, 1 out]
              }
            }
          }
          event User Event {
            n155 = event-data() -> ("ModuleID"=w300:i32, "Data"=w298:variant)  [unwired: 1 in]
            n156 = call <userlib>:"AddressedToThisModule.vi"("ModuleID"=w300, "ModuleAdmin"=w301) -> ("AddressedToThisInstance?"=w299:bool)  [unwired: 8 in, 1 out]
            n157 = case shown="True" w299 {
              tunnel: w296 -> [_ w305]
              tunnel: w298 -> [_ _]
              tunnel: [_ w303] -> w297
              frame False {
              }
              frame True {
                w304 = "StartData" ("State In")
                n158 = call "SetGetState.vi"("Set (f)"=TRUE, "State In"=w304) -> ()  [unwired: 9 in, 1 out]
                n159 = call "Enqueue.vi"("Enum"=enum16{"Else", "LE"}."LE", "Message"=w304, "MessageQueue"=w305) -> ("error out"=w303:errorcluster)  [unwired: 7 in, 1 out]
              }
            }
          }
          event User Event {
            n160 = event-data() -> ("ModuleID"=w311:i32, "Data"=w309:variant)  [unwired: 1 in]
            n161 = call <userlib>:"AddressedToThisModule.vi"("ModuleID"=w311, "ModuleAdmin"=w312) -> ("AddressedToThisInstance?"=w310:bool)  [unwired: 8 in, 1 out]
            n162 = case shown="True" w310 {
              tunnel: w307 -> [_ w316]
              tunnel: w309 -> [_ _]
              tunnel: [_ w315] -> w308
              frame False {
              }
              frame True {
                w314 = "StopData" ("State In")
                n163 = call "SetGetState.vi"("Set (f)"=TRUE, "State In"=w314) -> ()  [unwired: 9 in, 1 out]
                n164 = call "Enqueue.vi"("Enum"=enum16{"Else", "LE"}."LE", "Message"=w314, "MessageQueue"=w316) -> ("error out"=w315:errorcluster)  [unwired: 7 in, 1 out]
              }
            }
          }
        }
        n165 = call "ErrorHandler.vi"("error in (no error)"=w192, "MessageQueue"=w190) -> ("error out"=w191:errorcluster)  [unwired: 8 in, 1 out]
      }
      n166 = while {
        tunnel: w61 -> [w79]
        tunnel: w65 -> [w83]
        tunnel: [w82] -> w64
        tunnel: w63 -> [w80]
        tunnel: w59 -> [w77]
        tunnel: w60 -> [w74]
        stop <- w84 stop-if-true
        # "Sensor Producer Loop (SPL)"
        n167 = call "SetGetState.vi"() -> ("State Out"=w85:string)  [unwired: 11 in]
        n168 = call "Dequeue.vi"("Preview Queue (F)"=TRUE ("Preview Queue"), "error in (no error)"=w79, "MessageQueue"=w77) -> ("error out"=w78:errorcluster, "Message"=w73:string, "MessageQueue"=w76:refnum<queue>)  [unwired: 5 in, 1 out]
        n169 = case shown="\"StartData\"" w73 {
          tunnel: [_ _ _ _ _ TRUE] -> w84
          tunnel: [w89 w93 w104 w128 w167 w187] -> w81
          tunnel: w78 -> [w90 w93 w98 w130 w172 w187]
          tunnel: w80 -> [_ _ w103 w129 w170 _]
          tunnel: w76 -> [w88 _ w101 w120 w165 _]
          tunnel: w74 -> [_ _ w99 w121 w162 _]
          tunnel: w85 -> [_ _ _ _ _ _]
          frame "Init" {
            w87 = "Idle" ("State In")
            n170 = call "SetGetState.vi"("Set (f)"=TRUE, "State In"=w87) -> ()  [unwired: 9 in, 1 out]
            n171 = call "Enqueue.vi"("Enum"=enum16{"Else", "LE"}."LE", "error in (no error)"=w90, "Message"=w87, "MessageQueue"=w88) -> ("error out"=w89:errorcluster)  [unwired: 6 in, 1 out]
          }
          frame "Idle", Default {
            n172 = Wait (ms)(milliseconds to wait=u32 10) -> ()  [unwired: 1 out]
          }
          frame "StartData" {
            w100 = "Run" ("State In")
            n173 = disable-structure shown="Enabled" {
              disable-tunnel: w98 -> [w108 w116]
              disable-tunnel: [w107 w114] -> w97
              disable-tunnel: w99 -> [_ w118]
              frame Disabled {
                n174 = call "SetGetClass.vi"() -> ("Class Out"=w111:refnum<class "SensorBase.lvclass">)  [unwired: 11 in]
                n175 = call-dynamic "StartData.vi"("error in (no error)"=w108, "Class In"=w111) -> ("error out"=w107:errorcluster, "Class Out"=w110:refnum<class "SensorBase.lvclass">)  [unwired: 8 in]
                n176 = call "SetGetClass.vi"("Set (f)"=TRUE, "Class In"=w110) -> ()  [unwired: 9 in, 1 out]
              }
              frame Enabled {
                n177 = Preview Queue Element(queue=w118, error in (no error)=w116) -> (queue out=w113:refnum<queue>, element=w117:refnum<class "SensorBase.lvclass">, error out=w119:errorcluster)  [unwired: 1 in, 1 out]
                n178 = call-dynamic "StartData.vi"("error in (no error)"=w119, "Class In"=w117) -> ("error out"=w115:errorcluster, "Class Out"=w112:refnum<class "SensorBase.lvclass">)  [unwired: 8 in]
                n179 = Lossy Enqueue Element(queue=w113, element=w112, error in (no error)=w115) -> (error out=w114:errorcluster)  [unwired: 3 out]
              }
            }
            n180 = call "SetGetState.vi"("Set (f)"=TRUE, "State In"=w100) -> ()  [unwired: 9 in, 1 out]
            n181 = call "Enqueue.vi"("Enum"=enum16{"Else", "LE"}."LE", "error in (no error)"=w97, "Message"=w100, "MessageQueue"=w101) -> ("error out"=w96:errorcluster)  [unwired: 6 in, 1 out]
            n182 = property class="ModuleAdmin.lvclass"(reference=w103, error in=w96) -> (error out=w95:errorcluster, "Accessors:Module ID"=w102:i32)  [unwired: 1 out]
            n183 = call "StatusUpdate.vi"("error in (no error)"=w95, "Status"="Data Started", "ModuleID"=w102) -> ("error out"=w104:errorcluster)  [unwired: 8 in]
          }
          frame "Run" {
            n184 = disable-structure shown="Enabled" {
              disable-tunnel: w130 -> [w134 w141]
              disable-tunnel: [w133 w138] -> w127
              disable-tunnel: [w132 w142] -> w126
              disable-tunnel: [w131 w139] -> w124
              disable-tunnel: w121 -> [_ w140]
              frame Disabled {
                n185 = call "SetGetClass.vi"() -> ("Class Out"=w137:refnum<class "SensorBase.lvclass">)  [unwired: 11 in]
                n186 = call-dynamic "Run.vi"("error in (no error)"=w134, "SensorBase in"=w137) -> ("error out"=w132:errorcluster, "DataValid"=w131:bool, "clSensorData"=w133:T5, "SensorBase out"=w136:refnum<class "SensorBase.lvclass">)  [unwired: 6 in]
                n187 = call "SetGetClass.vi"("Set (f)"=TRUE, "Class In"=w136) -> ()  [unwired: 9 in, 1 out]
              }
              frame Enabled {
                n188 = Preview Queue Element(queue=w140, error in (no error)=w141) -> (queue out=w147:refnum<queue>, element=w143:refnum<class "SensorBase.lvclass">, error out=w146:errorcluster)  [unwired: 1 in, 1 out]
                n189 = call-dynamic "Run.vi"("error in (no error)"=w146, "SensorBase in"=w143) -> ("error out"=w145:errorcluster, "DataValid"=w139:bool, "clSensorData"=w138:T5, "SensorBase out"=w144:refnum<class "SensorBase.lvclass">)  [unwired: 6 in]
                n190 = Lossy Enqueue Element(queue=w147, element=w144, error in (no error)=w145) -> (error out=w142:errorcluster)  [unwired: 3 out]
              }
            }
            n191 = Unbundle By Name(w126) -> ("status"=w125:bool)
            n192 = Not(x=w125) -> (.not. x?=w122:bool)
            n193 = And(x=w122, y=w124) -> (x .and. y?=w123:bool)
            n194 = case shown="False" w123 {
              tunnel: w129 -> [_ w160]
              tunnel: [w152 w159] -> w128
              tunnel: w127 -> [_ w157]
              tunnel: w126 -> [w153 w156]
              tunnel: w120 -> [w151 _]
              frame False {
                w149 = "StopData" ("State In")
                n195 = call "SetGetState.vi"("Set (f)"=TRUE, "State In"=w149) -> ()  [unwired: 9 in, 1 out]
                n196 = call "Enqueue.vi"("Enum"=enum16{"Else", "LE"}."LE", "Priority (F)"=TRUE, "error in (no error)"=w153, "Message"=w149, "MessageQueue"=w151) -> ("error out"=w152:errorcluster)  [unwired: 5 in, 1 out]
              }
              frame True {
                n197 = property class="ModuleAdmin.lvclass"(reference=w160, error in=w156) -> (error out=w155:errorcluster, "Accessors:Module ID"=w158:i32)  [unwired: 1 out]
                n198 = call "SensorReport.vi"("ModuleID"=w158, "error in (no error)"=w155, "clSensorData"=w157) -> ("error out"=w159:errorcluster)  [unwired: 8 in]
              }
            }
          }
          frame "StopData" {
            w166 = "Idle" ("State In")
            n199 = disable-structure shown="Enabled" {
              disable-tunnel: w172 -> [w178 w182]
              disable-tunnel: [w174 w181] -> w164
              disable-tunnel: w162 -> [_ w179]
              frame Disabled {
                n200 = call "SetGetClass.vi"() -> ("Class Out"=w177:refnum<class "SensorBase.lvclass">)  [unwired: 11 in]
                n201 = call-dynamic "StopData.vi"("error in (no error)"=w178, "Class In"=w177) -> ("error out"=w174:errorcluster, "Class Out"=w176:refnum<class "SensorBase.lvclass">)  [unwired: 8 in]
                n202 = call "SetGetClass.vi"("Set (f)"=TRUE, "Class In"=w176) -> ()  [unwired: 9 in, 1 out]
              }
              frame Enabled {
                n203 = Preview Queue Element(queue=w179, error in (no error)=w182) -> (queue out=w183:refnum<queue>, element=w186:refnum<class "SensorBase.lvclass">, error out=w185:errorcluster)  [unwired: 1 in, 1 out]
                n204 = call-dynamic "StopData.vi"("error in (no error)"=w185, "Class In"=w186) -> ("error out"=w184:errorcluster, "Class Out"=w180:refnum<class "SensorBase.lvclass">)  [unwired: 8 in]
                n205 = Lossy Enqueue Element(queue=w183, element=w180, error in (no error)=w184) -> (error out=w181:errorcluster)  [unwired: 3 out]
              }
            }
            n206 = property class="ModuleAdmin.lvclass"(reference=w170, error in=w164) -> (error out=w163:errorcluster, "Accessors:Module ID"=w169:i32)  [unwired: 1 out]
            n207 = call "StatusUpdate.vi"("error in (no error)"=w163, "Status"="Data Stopped", "ModuleID"=w169) -> ("error out"=w168:errorcluster)  [unwired: 8 in]
            n208 = call "SetGetState.vi"("Set (f)"=TRUE, "State In"=w166) -> ()  [unwired: 9 in, 1 out]
            n209 = call "Enqueue.vi"("Enum"=enum16{"Else", "LE"}."LE", "error in (no error)"=w168, "Message"=w166, "MessageQueue"=w165) -> ("error out"=w167:errorcluster)  [unwired: 6 in, 1 out]
          }
          frame "Exit" {
          }
        }
        n210 = call "ErrorHandler.vi"("error in (no error)"=w81, "MessageQueue"=w83) -> ("error out"=w82:errorcluster)  [unwired: 8 in, 1 out]
      }
    }
    frame Error {
      w608 = T6 2 items=["no dialog", "OK message", "continue or stop message", "OK message + warnings", "continue/stop + warnings"] ("type of dialog (OK msg:1)")
      n211 = property class="ModuleAdmin.lvclass"(reference=w615) -> (reference out=w613:refnum<class "ModuleAdmin.lvclass">, error out=w609:errorcluster, "Accessors:CloneRegRef"=w612:refnum<data-value>, "Accessors:Module ID"=w611:i32)  [unwired: 1 in]
      n212 = call <userlib>:"Remove.vi"("error in (no error)"=w609, "Module ID"=w611, "CloneRegRef"=w612) -> ("error out"=w617:errorcluster)  [unwired: 6 in, 2 out]
      n213 = flat-sequence {
        tunnel: w618 -> [w621]
        tunnel: w617 -> [_]
        tunnel: [w620] -> w616
        tunnel: w608 -> [w619]
        frame #0 {
          n214 = call <vilib>:"Simple Error Handler.vi"("type of dialog (OK msg:1)"=w619, "error in (no error)"=w621) -> ("error out"=w620:errorcluster)  [unwired: 3 in, 4 out]
        }
      }
    }
  }
  n215 = call "DestroyClone.vi"("error in (no error)"=w45, "Exit via Stop Module Req?"=w41, "Wait for Module to stop?"=w42, "ModuleAdmin"=w43) -> ("error out"=w44:errorcluster, "External Launch"=w40:bool)  [unwired: 5 in, 1 out]
  n216 = Unregister For Events(event registration refnum=w38, error in=w39) -> (error out=w37:errorcluster)
  n217 = Release Queue(queue=w50, force destroy? (F)=w2, error in (no error)=w44) -> (error out=w7:errorcluster)  [unwired: 2 out]
  n218 = Release Queue(queue=w4, force destroy? (F)=w2, error in (no error)=w7) -> (error out=w6:errorcluster)  [unwired: 2 out]
  n219 = Release Queue(queue=w3, force destroy? (F)=w2, error in (no error)=w6) -> (error out=w5:errorcluster)  [unwired: 2 out]
  n220 = Merge Errors(w37, w5, w19) -> (w29:errorcluster)
  n221 = case shown="True" w40 {
    tunnel: w29 -> [w622 w625]
    tunnel: [w622 w623] -> w28
    frame False {
    }
    frame True {
      n222 = control-ref of="This VI"() -> (w624:refnum<vi>)
      n223 = case shown="No Error" w625 {
        selector: w625 -> [w627 _]
        tunnel: w624 -> [w628 w630]
        tunnel: [w626 w629] -> w623
        frame No Error {
          n224 = invoke class="VI" method="FP.Close"(reference=w628, error in=w627) -> (error out=w626:errorcluster)  [unwired: 1 in, 2 out]
        }
        frame Error {
          n225 = invoke class="VI" method="FP.Open"(reference=w630, "Activate"=TRUE ("Activate?")) -> (error out=w629:errorcluster)  [unwired: 3 in, 4 out]
        }
      }
    }
  }
  "error out" <- w28
